vi "4Pi Capture Scan Counter 1.vi"(8 "Scan Tracker":T1) -> (0 "Scan Tracker Out":T1, 1 "To cycle?":bool, 2 "Move stage?":bool, 3 "Exit?":bool)   [LabVIEW 2016]
uses:
  4Pi Capture Manager Controls/4Pi Capture Scan Tracker.ctl
  4Pi Capture Manager Controls/4Pi Capture Switch Laser.ctl
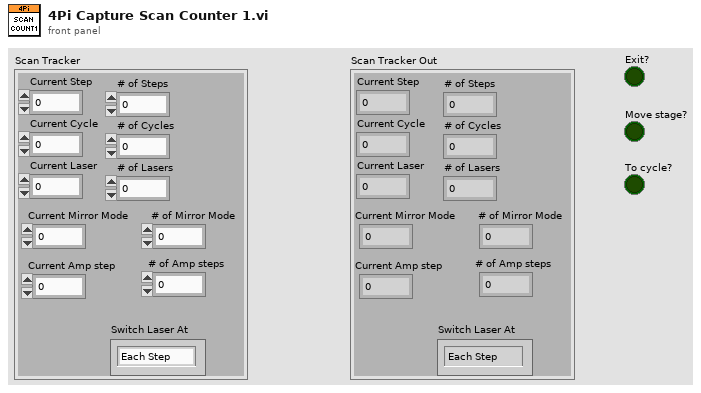
[diagram p1: front panel]
types:
  T1 = typedef "4Pi Capture Scan Tracker.ctl" = cluster{"Current Step":u16, "Current Cycle":u16, "Current Laser":u16, "# of Lasers":u16, "# of Cycles":u16, "# of Steps":u16, "Switch Laser At":T2, "Current Mirror Mode":u16, "# of Mirror Mode":u16, "Current Amp step":u16, "# of Amp steps":u16}
  T2 = typedef "4Pi Capture Switch Laser.ctl" = enum16{"Each Step", "Each Cycle", "All Cycles"}
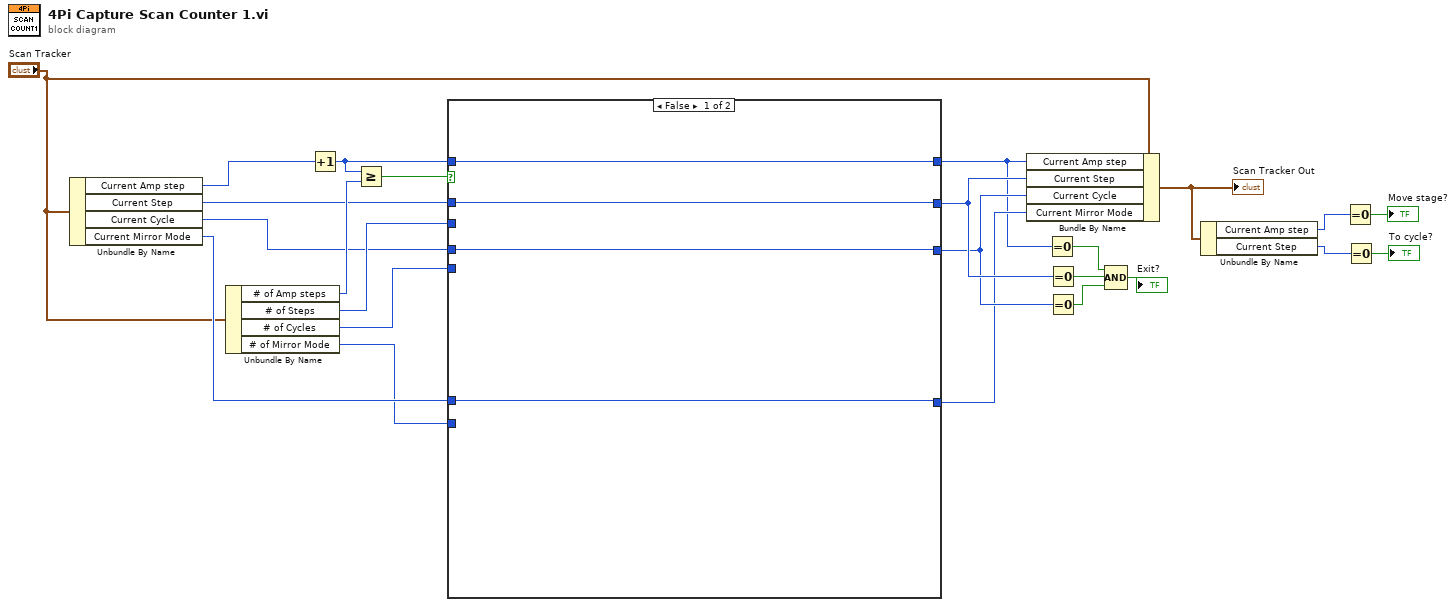
[diagram p0: block diagram]
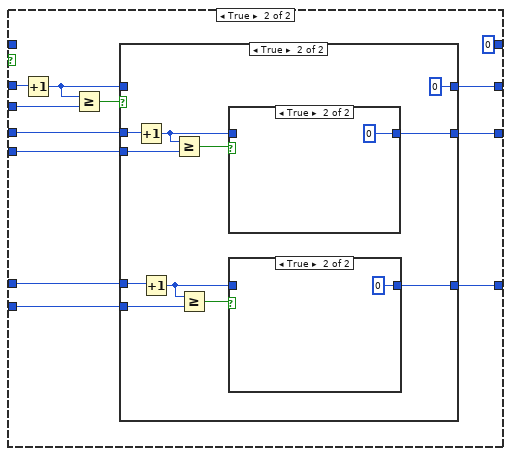
[diagram p2: hidden frame]
diagram:
  n1 = Unbundle By Name("Scan Tracker") -> ("Current Amp step"=w24:u16, "Current Step"=w20:u16, "Current Cycle"=w18:u16, "Current Mirror Mode"=w16:u16)
  n2 = Unbundle By Name("Scan Tracker") -> ("# of Amp steps"=w23:u16, "# of Steps"=w19:u16, "# of Cycles"=w17:u16, "# of Mirror Mode"=w15:u16)
  n3 = Increment(x=w24) -> (x+1=w22:u16)
  n4 = Greater Or Equal?(x=w22, y=w23) -> (x >= y?=w21:bool)
  n5 = case shown="False" w21 {
    tunnel: w22 -> [w28 _]
    tunnel: w20 -> [w27 w40]
    tunnel: w19 -> [_ w38]
    tunnel: [w28 u16 0] -> w1
    tunnel: [w27 w35] -> w13
    tunnel: w18 -> [w26 w34]
    tunnel: w17 -> [_ w33]
    tunnel: [w26 w32] -> w12
    tunnel: w16 -> [w25 w31]
    tunnel: w15 -> [_ w30]
    tunnel: [w25 w29] -> w11
    frame False {
    }
    frame True {
      n6 = Increment(x=w40) -> (x+1=w39:u16)
      n7 = Greater Or Equal?(x=w39, y=w38) -> (x >= y?=w37:bool)
      n8 = case shown="True" w37 {
        tunnel: w39 -> [w43 _]
        tunnel: [w43 u16 0] -> w35
        tunnel: w34 -> [w42 w53]
        tunnel: w33 -> [_ w52]
        tunnel: [w42 w49] -> w32
        tunnel: w31 -> [w41 w48]
        tunnel: w30 -> [_ w46]
        tunnel: [w41 w44] -> w29
        frame False {
        }
        frame True {
          n9 = Increment(x=w53) -> (x+1=w51:u16)
          n10 = Increment(x=w48) -> (x+1=w47:u16)
          n11 = Greater Or Equal?(x=w51, y=w52) -> (x >= y?=w50:bool)
          n12 = Greater Or Equal?(x=w47, y=w46) -> (x >= y?=w45:bool)
          n13 = case shown="True" w50 {
            tunnel: w51 -> [w57 _]
            tunnel: [w57 u16 0] -> w49
            frame False {
            }
            frame True {
            }
          }
          n14 = case shown="True" w45 {
            tunnel: w47 -> [w55 _]
            tunnel: [w55 u16 0] -> w44
            frame False {
            }
            frame True {
            }
          }
        }
      }
    }
  }
  n15 = Bundle By Name(cluster="Scan Tracker", "Current Amp step"=w1, "Current Step"=w13, "Current Cycle"=w12, "Current Mirror Mode"=w11) -> (w7:T1)
  "Scan Tracker Out" <- w7
  n16 = Equal To 0?(x=w1) -> (x = 0?=w2:bool)
  n17 = Equal To 0?(x=w13) -> (x = 0?=w10:bool)
  n18 = Equal To 0?(x=w12) -> (x = 0?=w9:bool)
  n19 = Compound Arithmetic op=AND(w2, w10, w9) -> (→"Exit?":bool)
  n20 = Unbundle By Name(w7) -> ("Current Amp step"=w6:u16, "Current Step"=w4:u16)
  n21 = Equal To 0?(x=w6) -> (x = 0?=→"Move stage?":bool)
  n22 = Equal To 0?(x=w4) -> (x = 0?=→"To cycle?":bool)
